vi "Recognizing Vision Target.vi"(4 "Image Src":T1) -> (0 "Distance (ft)":dbl, 1 "Boolean":bool, 2 "Angle 2":dbl)   [LabVIEW 2018]
uses:
  <vilib>/vision/Image Controls.llb/IMAQ Image.ctl
  Vision/Camera Types.ctl
  <vilib>/vision/NI_Vision_Development_Module.lvlib
panel:
  out "Array":T2(array[cluster])
  out "Image 5":T1(plugin-control)
  out "Particles 2":i32
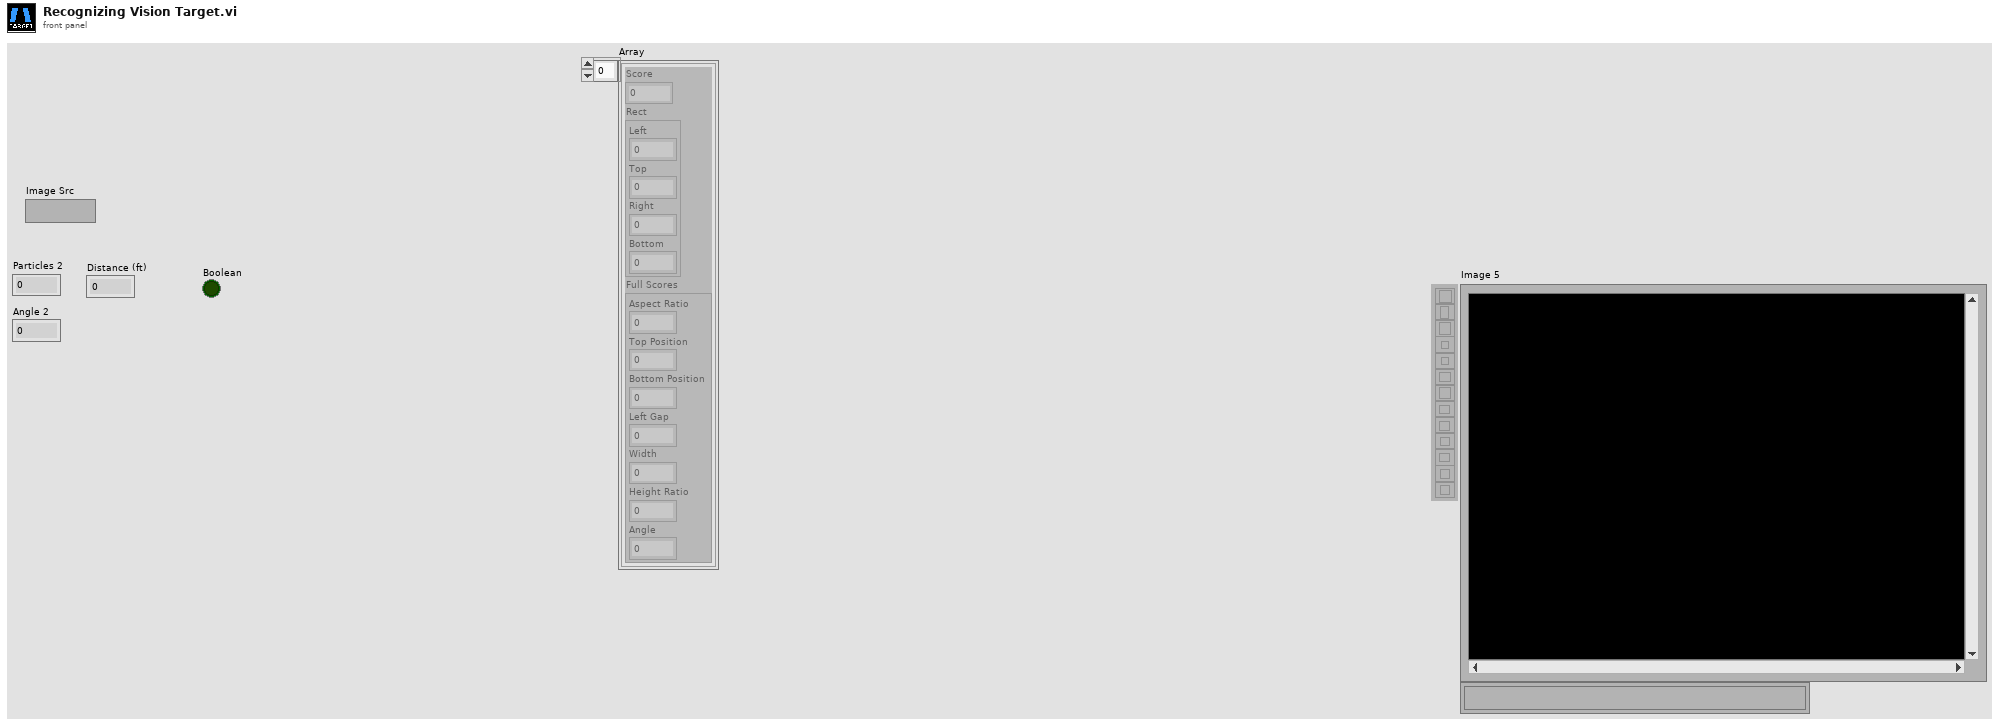
[diagram p1: front panel]
types:
  T1 = typedef "IMAQ Image.ctl" = refnum<image>
  T2 = cluster{"Score":dbl, "Rect":cluster{"Left":dbl, "Top":dbl, "Right":dbl, "Bottom":dbl}, "Full Scores":cluster{"Aspect Ratio":dbl, "Top Position":dbl, "Bottom Position":dbl, "Left Gap":dbl, "Width":dbl, "Height Ratio":dbl, "Angle":dbl}}[]
  T3 = typedef "Particle Parameters" = i32
  T4 = typedef "Camera Types.ctl" = enum16{"206", "1011", "1013", "MS HD3000 square", "MS HD3000 640x480"}
  T5 = cluster{"Score":dbl, "Rect":cluster{"Left":dbl, "Top":dbl, "Right":dbl, "Bottom":dbl}, "Full Scores":cluster{"Aspect Ratio":dbl, "Top Position":dbl, "Bottom Position":dbl, "Left Gap":dbl, "Width":dbl, "Height Ratio":dbl, "Angle":dbl}}
  T6 = cluster{"Left":dbl, "Top":dbl, "Right":dbl, "Bottom":dbl}
  T7 = cluster{"Numeric":dbl, "Numeric":dbl, "Numeric":dbl, "Numeric":dbl}
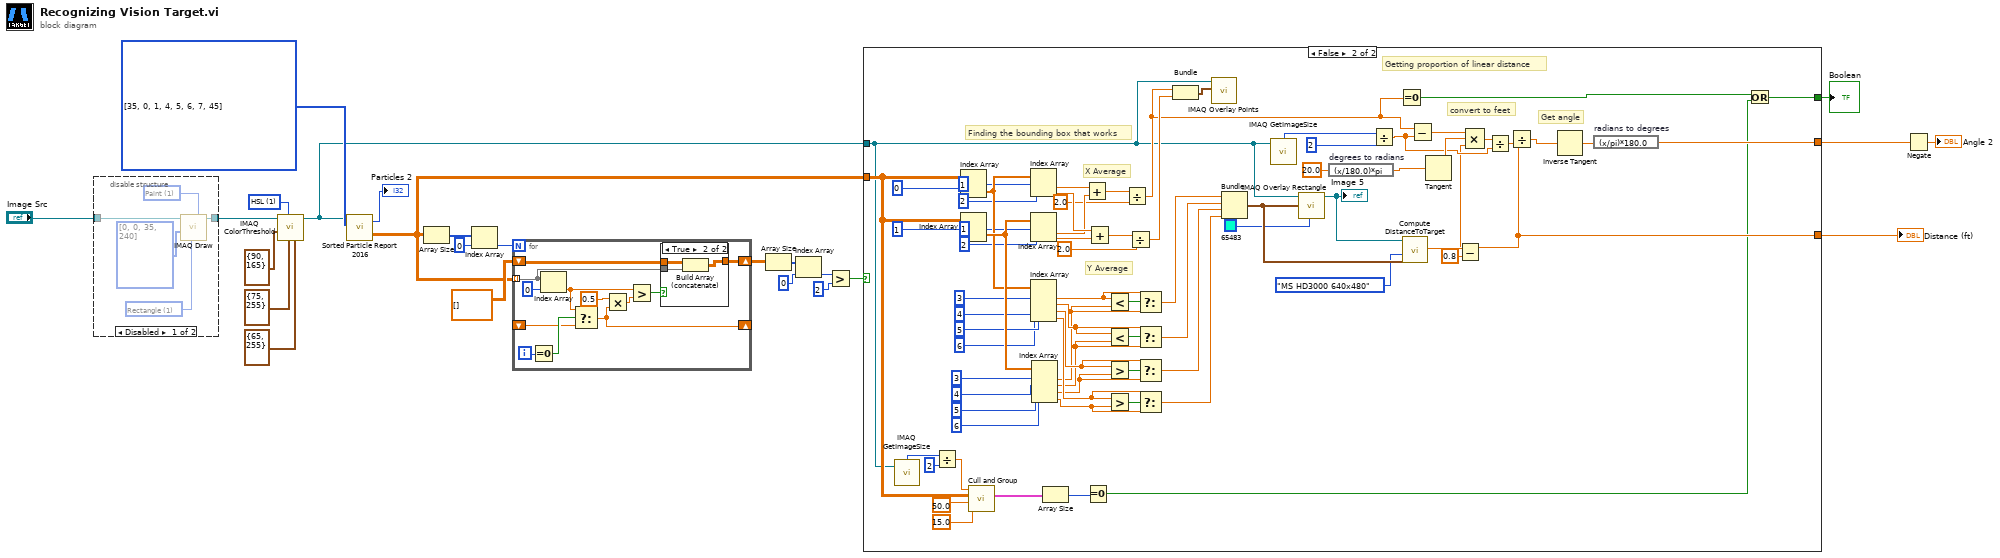
[diagram p0: block diagram]
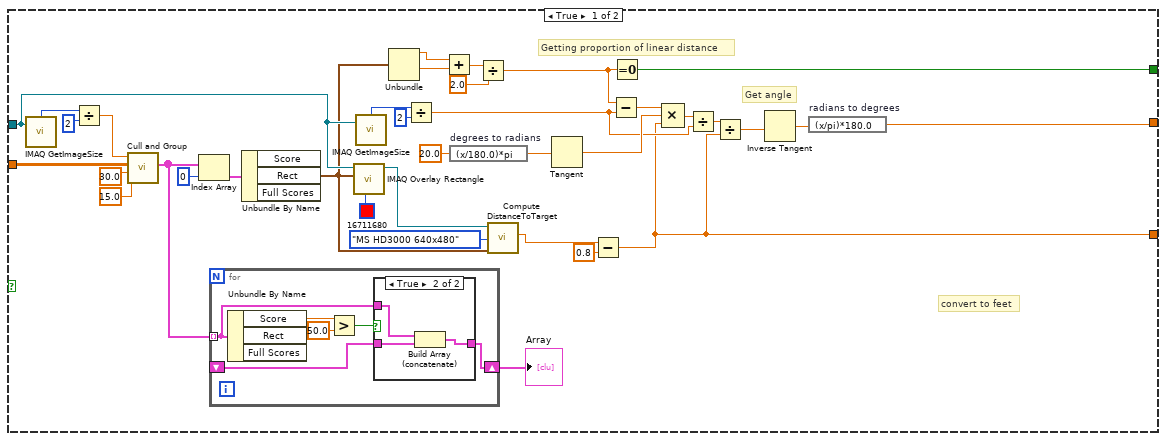
[diagram p3: hidden frame]
diagram:
  w4 = u16 1 items=["RGB", "HSL", "HSV", "HSI"] ("Color Mode")
  w23 = T3[] [35, 0, 1, 4, 5, 6, 7, 45] items=["Center of Mass X", "Center of Mass Y", "First Pixel X", "First Pixel Y", "Bounding Rect Left", "Bounding Rect Top", "Bounding Rect Right", "Bounding Rect Bottom", "Max Feret Diameter Start X", "Max Feret Diameter Start Y", "Max Feret Diameter End X", "Max Feret Diameter End Y", "Max Horiz. Segment Length Left", "Max Horiz. Segment Length Right", "Max Horiz. Segment Length Row", "-", "Bounding Rect Width", "Bounding Rect Height", "Bounding Rect Diagonal", "Perimeter", "Convex Hull Perimeter", "Holes' Perimeter", "Max Feret Diameter", "Equivalent Ellipse Major Axis", "Equivalent Ellipse Minor Axis", "Equivalent Ellipse Minor Axis (Feret)", "Equivalent Rect Long Side", "Equivalent Rect Short Side", "Equivalent Rect Diagonal", "Equivalent Rect Short Side (Feret)", "Average Horiz. Segment Length", "Average Vert. Segment Length", "Hydraulic Radius", "Waddel Disk Diameter", "-", "Area", "Holes' Area", "Particle & Holes' Area", "Convex Hull Area", "Image Area", "-", "Number of Holes", "Number of Horiz. Segments", "Number of Vert. Segments", "-", "Orientation", "Max Feret Diameter Orientation", "-", "% Area/Image Area", "% Area/(Particle & Holes' Area)", "Ratio of Equivalent Ellipse Axes", "Ratio of Equivalent Rect Sides", "-", "Elongation Factor", "Compactness Factor", "Heywood Circularity Factor", "Type Factor", "-", "Sum X", "Sum Y", "Sum XX", "Sum XY", "Sum YY", "Sum XXX", "Sum XXY", "Sum XYY", "Sum YYY", "-", "Moment of Inertia XX", "Moment of Inertia XY", "Moment of Inertia YY", "Moment of Inertia XXX", "Moment of Inertia XXY", "Moment of Inertia XYY", "Moment of Inertia YYY", "Norm. Moment of Inertia XX", "Norm. Moment of Inertia XY", "Norm. Moment of Inertia YY", "Norm. Moment of Inertia XXX", "Norm. Moment of Inertia XXY", "Norm. Moment of Inertia XYY", "Norm. Moment of Inertia YYY", "Hu Moment 1", "Hu Moment 2", "Hu Moment 3", "Hu Moment 4", "Hu Moment 5", "Hu Moment 6", "Hu Moment 7"] ("Pixel Measurements")
  n1 = disable-structure shown="Disabled" {
    disable-tunnel: "Image Src" -> [w29 w30]
    disable-tunnel: [w28 w30] -> w10
    frame Disabled {
      w26 = u16 1 items=["Frame", "Paint", "Invert Frame", "Invert Paint"] ("Draw Mode")
      w27 = u16 1 items=["Line", "Rectangle", "Oval"] ("Shape to draw")
      n2 = call "IMAQ Draw"("Draw Mode"=w26, "Shape to draw"=w27, "Coordinates"=i32[] [0, 0, 35, 240], "Image Src"=w29) -> ("Image Dst Out"=w28:T1)  [unwired: 6 in, 1 out]
    }
    frame Enabled {
    }
  }
  n3 = call "IMAQ ColorThreshold"("Blue or Luma or Val or Inten Range"=cluster{"Lower value":i32, "Upper value":i32} {"Lower value"=65, "Upper value"=255}, "Green or Sat Range"=cluster{"Lower value":i32, "Upper value":i32} {"Lower value"=75, "Upper value"=255}, "Color Mode"=w4, "Red or Hue Range"=cluster{"Lower value":i32, "Upper value":i32} {"Lower value"=90, "Upper value"=165}, "Image Src"=w10) -> ("Image Dst Out"=w11:T1)  [unwired: 5 in, 1 out]
  n4 = call "Sorted Particle Report 2016.vi"("Pixel Measurements"=w23, "Image in"=w11) -> ("Sorted Data"=w12:dbl[][], "Particles"=→"Particles 2":i32)  [unwired: 2 in]
  n5 = Array Size(array=w12) -> (size(s)=w17:i32[])
  n6 = Index Array(array=w17, index=0) -> (element=w15:i32)
  n7 = for {
    N: w15 -> [_]
    tunnel: w12 -> [w34] mode=indexing
    shift-right: [w38] -> _
    shift-left: _ -> [w39]
    shift-right: [w32] -> w14
    shift-left: dbl[][] [] -> [w33]
    i -> [w42]
    n8 = Equal To 0?(x=w42) -> (x = 0?=w40:bool)
    n9 = Index Array(array=w34, index=0) -> (element=w35:dbl)
    n10 = Select(t=w35, s=w40, f=w39) -> (s? t:f=w38:dbl)
    n11 = Multiply(x=0.5, y=w38) -> (x*y=w36:dbl)
    n12 = Greater?(x=w35, y=w36) -> (0:w31:bool)
    n13 = case shown="True" w31 {
      tunnel: w34 -> [_ w46]
      tunnel: w33 -> [w43 w45]
      tunnel: [w43 w44] -> w32
      frame False {
      }
      frame True {
        n14 = Build Array (concatenate)(w45, w46) -> (w44:dbl[][])
      }
    }
  }
  n15 = Array Size(array=w14) -> (size(s)=w20:i32[])
  n16 = Index Array(array=w20, index=0 ("y")) -> (element=w18:i32)
  n17 = Greater?(x=w18, y=2) -> (0:w13:bool)
  n18 = case shown="False" w13 {
    tunnel: w11 -> [w70 w93]
    tunnel: w12 -> [w80 w104]
    tunnel: [w47 w107] -> w7
    tunnel: [w62 w109] -> w8
    tunnel: [w52 w96] -> w6
    frame True {
      # "convert to feet"
      # "Get angle"
      # "Getting proportion of linear distance"
      n19 = call "IMAQ GetImageSize"("Image"=w70) -> ("X Resolution"=w76:i32)  [unwired: 3 in, 2 out]
      n20 = Divide(x=w76, y=2) -> (x/y=w74:dbl)
      n21 = call "Cull and Group.vi"("Min Compnt %"=15.0, "Score Cutoff %"=30.0, "Sorted Data"=w80, "Image Center"=w74) -> ("Best Targets above cutoff"=w51:T2)  [unwired: 7 in]
      n22 = Index Array(array=w51, index=0) -> (element=w81:T5)
      n23 = for {
        tunnel: w51 -> [w85] mode=indexing
        shift-right: [w84] -> w50
        shift-left: _ -> [w83]
        n24 = Unbundle By Name(w85) -> ("Score"=w88:dbl)  [unwired: 2 out]
        n25 = Greater?(x=w88, y=50.0) -> (0:w86:bool)
        n26 = case shown="True" w86 {
          tunnel: w85 -> [_ w91]
          tunnel: [w89 w92] -> w84
          tunnel: w83 -> [w89 w90]
          frame False {
          }
          frame True {
            n27 = Build Array (concatenate)(w91, w90) -> (w92:T2)
          }
        }
      }
      "Array" <- w50
      n28 = Unbundle By Name(w81) -> ("Rect"=w64:T6)  [unwired: 2 out]
      n29 = call "IMAQ Overlay Rectangle"("Color"=u32 16711680, "Rectangle"=w64, "Image"=w70) -> ("Image Out"=w63:T1)  [unwired: 7 in, 1 out]
      n30 = call "IMAQ GetImageSize"("Image"=w70) -> ("X Resolution"=w73:i32)  [unwired: 3 in, 2 out]
      n31 = Unbundle(w64) -> ("Left"=w69:dbl, "Right"=w68:dbl)  [unwired: 2 out]
      n32 = Divide(x=w73, y=2) -> (x/y=w55:dbl)
      n33 = Add(x=w69, y=w68) -> (x+y=w66:dbl)
      n34 = expression code="(x/180.0)*pi" "degrees to radians"(20.0) -> (w56:dbl)
      n35 = Divide(x=w66, y=2.0) -> (x/y=w53:dbl)
      n36 = call "Compute DistanceToTarget.vi"("Rect"=w64, "Camera Type"=Camera_Types."MS HD3000 640x480", "Image Src"=w63) -> ("Distance (ft)"=w48:dbl)  [unwired: 7 in, 1 out]
      n37 = Tangent(1:w56) -> (0:w60:dbl)
      n38 = Subtract(x=w48, y=0.8) -> (x-y=w47:dbl)
      n39 = Subtract(x=w53, y=w55) -> (x-y=w61:dbl)
      n40 = Equal To 0?(x=w53) -> (x = 0?=w52:bool)
      n41 = Compound Arithmetic op=MULTIPLY(w61, w60, w47) -> (w59:dbl)
      n42 = Divide(x=w59, y=w55) -> (x/y=w58:dbl)
      n43 = Divide(x=w58, y=w47) -> (x/y=w54:dbl)
      n44 = Inverse Tangent(1:w54) -> (0:w72:dbl)
      n45 = expression code="(x/pi)*180.0" "radians to degrees"(w72) -> (w62:dbl)
    }
    frame False {
      # "convert to feet"
      # "Get angle"
      # "Getting proportion of linear distance"
      # "Finding the bounding box that works"
      # "Y Average"
      # "X Average"
      n46 = call "IMAQ GetImageSize"("Image"=w93) -> ("X Resolution"=w100:i32)  [unwired: 3 in, 2 out]
      n47 = Divide(x=w100, y=2) -> (x/y=w99:dbl)
      n48 = Index Array(array=w104, index (row)=0) -> (element=w146:dbl[])  [unwired: 1 in]
      n49 = Index Array(array=w104, index (row)=1 ("disabled index (col)")) -> (element=w147:dbl[])  [unwired: 1 in]
      n50 = call "Cull and Group.vi"("Min Compnt %"=15.0, "Score Cutoff %"=50.0, "Sorted Data"=w104, "Image Center"=w99) -> ("Best Targets above cutoff"=w98:T2)  [unwired: 7 in]
      n51 = Index Array(array=w146, index #1=1 ("index"), index #2=2 ("index")) -> (element #1=w140:dbl, element #2=w142:dbl)
      n52 = Index Array(array=w147, index #1=1 ("index"), index #2=2 ("index")) -> (element #1=w141:dbl, element #2=w139:dbl)
      n53 = Index Array(array=w146, index #1=3 ("index"), index #2=4 ("index"), index #3=5 ("index"), index #4=6 ("index")) -> (element #1=w149:dbl, element #2=w153:dbl, element #3=w155:dbl, element #4=w158:dbl)
      n54 = Index Array(array=w147, index #1=3 ("index"), index #2=4 ("index"), index #3=5 ("index"), index #4=6 ("index")) -> (element #1=w150:dbl, element #2=w152:dbl, element #3=w156:dbl, element #4=w159:dbl)
      n55 = Array Size(array=w98) -> (size(s)=w97:i32)
      n56 = Add(x=w140, y=w141) -> (x+y=w137:dbl)
      n57 = Equal To 0?(x=w97) -> (x = 0?=w95:bool)
      n58 = Add(x=w142, y=w139) -> (x+y=w138:dbl)
      n59 = Less?(x=w149, y=w150) -> (x < y?=w148:bool)
      n60 = Less?(x=w153, y=w152) -> (x < y?=w151:bool)
      n61 = Greater?(x=w155, y=w156) -> (0:w154:bool)
      n62 = Greater?(x=w158, y=w159) -> (0:w157:bool)
      n63 = Divide(x=w137, y=2.0) -> (x/y=w116:dbl)
      n64 = Divide(x=w138, y=2.0) -> (x/y=w166:dbl)
      n65 = Select(t=w149, s=w148, f=w150) -> (s? t:f=w160:dbl)
      n66 = Select(t=w153, s=w151, f=w152) -> (s? t:f=w161:dbl)
      n67 = Select(t=w155, s=w154, f=w156) -> (s? t:f=w162:dbl)
      n68 = Select(t=w158, s=w157, f=w159) -> (s? t:f=w163:dbl)
      n69 = Bundle(w116, w166) -> (w165:cluster{dbl, dbl})  [unwired: 1 in]
      n70 = call "IMAQ Overlay Points"("Point"=w165, "Image"=w93) -> ()  [unwired: 8 in, 2 out]
      n71 = Bundle("Numeric"=w160, "Numeric"=w161, "Numeric"=w162, "Numeric"=w163) -> (w164:T7)  [unwired: 1 in]
      n72 = call "IMAQ GetImageSize"("Image"=w93) -> ("X Resolution"=w143:i32)  [unwired: 3 in, 2 out]
      n73 = call "IMAQ Overlay Rectangle"("Color"=u32 65483, "Rectangle"=w164, "Image"=w93) -> ("Image Out"=w145:T1)  [unwired: 7 in, 1 out]
      "Image 5" <- w145
      n74 = expression code="(x/180.0)*pi" "degrees to radians"(20.0 ("Numeric")) -> (w110:dbl)
      n75 = Divide(x=w143, y=2) -> (x/y=w112:dbl)
      n76 = Equal To 0?(x=w116) -> (x = 0?=w94:bool)
      n77 = call "Compute DistanceToTarget.vi"("Rect"=w164, "Camera Type"=Camera_Types."MS HD3000 640x480", "Image Src"=w145) -> ("Distance (ft)"=w108:dbl)  [unwired: 7 in, 1 out]
      n78 = Subtract(x=w116, y=w112) -> (x-y=w115:dbl)
      n79 = Tangent(1:w110) -> (0:w114:dbl)
      n80 = Subtract(x=w108, y=0.8) -> (x-y=w107:dbl)
      n81 = Compound Arithmetic op=MULTIPLY(w115, w114, w107) -> (w113:dbl)
      n82 = Divide(x=w113, y=w112) -> (x/y=w111:dbl)
      n83 = Divide(x=w111, y=w107) -> (x/y=w117:dbl)
      n84 = Inverse Tangent(1:w117) -> (0:w144:dbl)
      n85 = expression code="(x/pi)*180.0" "radians to degrees"(w144) -> (w109:dbl)
      n86 = Or(x=w94, y=w95) -> (x .or. y?=w96:bool)
    }
  }
  "Distance (ft)" <- w7
  "Boolean" <- w6
  n87 = Negate(x=w8) -> (-x=→"Angle 2":dbl)
